vi "PH_ImageCalibrator.write Energy Pic.vi"(0 "i ref in":refnum<vi>, 2 "Cam Image":T1, 5 "error in (no error)":errorcluster) -> (14 "i ref out":refnum<vi>, 19 "error out":errorcluster)   [LabVIEW 2014, in "PH_ImageCalibrator.lvlib"]
doc: "This VI adds the incoming Cam Image to the erngy image and sets the number of accumulated energy pics up by one."
uses:
  PH_ImageCalibrator.lvlib
  <vilib>/vision/Image Controls.llb/IMAQ Image.ctl
  CS_Core/BaseSM/BaseSM.lvlib
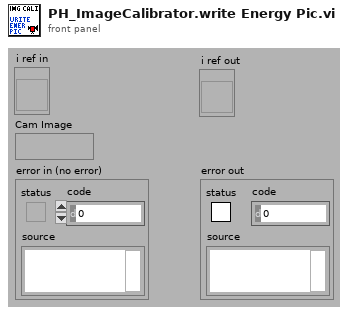
[diagram p1: front panel]
types:
  T1 = typedef "IMAQ Image.ctl" = refnum<image>
  T2 = typedef "PH_ImageCalibrator.lvlib/PH_ImageCalibrator.i attribute.ctl" = cluster{"GUI Refs":cluster{"Available Cams":refnum<vi>, "OK":refnum<vi>, "Skip":refnum<vi>, "Repeat":refnum<vi>, "Cancel":refnum<vi>, "Length [mm]":refnum<vi>, "Energy [mJ]":refnum<vi>, "Dialog":refnum<vi>}, "Cam instances":string[], "Dark Pics":cluster{"#":i32, "BI taken":bool}, "Lin Cali":cluster{"Distance [Pixel]":dbl, "Distance [mm]":dbl, "Lin Cali Factor [mm/Pixel]":dbl}, "Energy Cali":cluster{"Pixelsum":dbl, "Energy [mJ]":dbl, "Energy Cali factor [mJ/Pixelsum]":dbl, "Underground subtracted?":bool, "#":i32}, "Images":cluster{"Background":T1, "Energy":T1}}
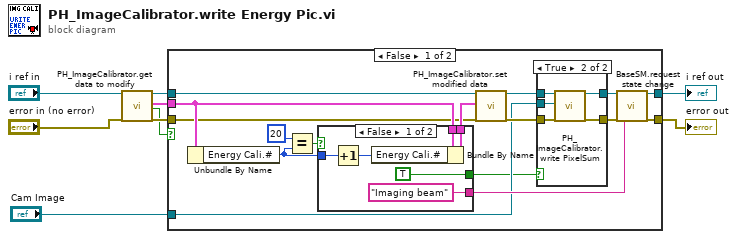
[diagram p0: block diagram]
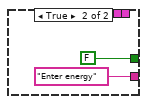
[diagram p3: hidden frame]
diagram:
  n1 = call "PH_ImageCalibrator.get data to modify.vi"("i ref in"="i ref in", "error in (no error)"="error in (no error)") -> ("i ref out"=w7:refnum<vi>, "i attribute"=w9:T2, "timed out"=w4:bool, "error out"=w5:errorcluster)  [unwired: 14 in]
  n2 = case shown="False" w4 {
    tunnel: w9 -> [w25 _]
    tunnel: [w22 w43] -> w8
    tunnel: w7 -> [w10 w43]
    tunnel: [w21 w42] -> w6
    tunnel: w5 -> [w11 w42]
    tunnel: "Cam Image" -> [w14 _]
    frame False {
      n3 = Unbundle By Name(w25) -> ("Energy Cali.#"=w24:i32)
      n4 = Equal?(x=20 ("# of wanted pics for energy calibration"), y=w24) -> (x = y?=w23:bool)
      n5 = case shown="False" w23 {
        tunnel: w25 -> [w37 w40]
        tunnel: w24 -> [w34 _]
        tunnel: ["Imaging beam" "Enter energy"] -> w20
        tunnel: [w35 w40] -> w19
        tunnel: [TRUE FALSE] -> w13
        frame False {
          n6 = Increment(x=w34) -> (x+1=w36:i32)
          n7 = Bundle By Name(cluster=w37, "Energy Cali.#"=w36) -> (w35:T2)
        }
        frame True {
        }
      }
      n8 = call "PH_ImageCalibrator.set modified data.vi"("i ref in"=w10, "i attribute"=w19, "error in (no error)"=w11) -> ("i ref out"=w18:refnum<vi>, "error out"=w16:errorcluster)  [unwired: 15 in]
      n9 = case shown="True" w13 {
        tunnel: w18 -> [w27 w32]
        tunnel: [w27 w31] -> w17
        tunnel: w16 -> [w26 w30]
        tunnel: [w26 w29] -> w15
        tunnel: w14 -> [_ w28]
        frame False {
        }
        frame True {
          n10 = call "PH_ImageCalibrator.write PixelSum.vi"("i ref in"=w32, "Cam Image"=w28, "error in (no error)"=w30) -> ("i ref out"=w31:refnum<vi>, "error out"=w29:errorcluster)  [unwired: 15 in]
        }
      }
      n11 = call "BaseSM.request state change.vi"("i ref in"=w17, "error in (no error)"=w15, "requested state"=w20) -> ("i ref out"=w22:refnum<vi>, "error out"=w21:errorcluster)  [unwired: 13 in, 2 out]
    }
    frame True {
    }
  }
  "i ref out" <- w8
  "error out" <- w6
